vi "平均计算FRF.vi"(0 "time signal X":waveform(dbl) caption="时间信号X", 1 "restart averaging (F)":bool caption="重新开始平均(F)", 2 "window parameter":dbl=nan caption="窗参数", 5 "time signal Y":waveform(dbl) caption="时间信号Y", 7 "window":T2=1 caption="窗" items=["矩形"=0, "Hanning"=1, "Hamming"=2, "Blackman-Harris"=3, "Exact Blackman"=4, "Blackman"=5, "Flat Top"=6, "4阶Blackman-Harris "=7, "7阶Blackman-Harris"=8, "Low Sidelobe"=9, "Blackman Nuttall"=11, "三角"=30, "Bartlett-Hanning"=31, "Bohman"=32, "Parzen"=33, "Welch"=34, "Kaiser"=60, "Dolph-Chebyshev"=61, "高斯"=62], 9 "view":T1 caption="查看", 11 "error in (no error)":errorcluster caption="错误输入（无错误）", 12 "averaging parameters":T3={"averaging mode"=enum."No averaging", "weighting mode"=enum."Exponential", "number of averages"=10} caption="平均参数" {"number of averages" min=1}, 13 "FRF Mode":enum16{"H1", "H2", "H3"}(ring) caption="FRF模式", 14 "删除上一波形":bool caption="删除上一次波形") -> (3 "averaging done":bool caption="完成平均", 4 "magnitude":cluster{"f0":dbl, "df":dbl, "magnitude":dbl[]} caption="幅度" {"magnitude" format="%.2p"; "f0" format="%0.2p"; "df" format="%0.2p"}, 6 "phase":cluster{"f0":dbl, "df":dbl, "phase":dbl[]} caption="相位" {"phase" format="%.2p"; "f0" format="%0.2p"; "df" format="%0.2p"}, 8 "coherence":cluster{"f0":dbl, "df":dbl, "coherence":dbl[]} caption="相关", 10 "averages completed":dbl caption="已完成平均数" format="%.2p", 15 "error out":errorcluster caption="错误输出")   [LabVIEW 2014]
uses:
  <vilib>/Analysis/4window.llb/windowTd.ctl
  <vilib>/measure/maspectr.llb/2-chan State.ctl
  <vilib>/measure/NI_MAPro.lvlib
  <vilib>/Analysis/NI_AALPro.lvlib
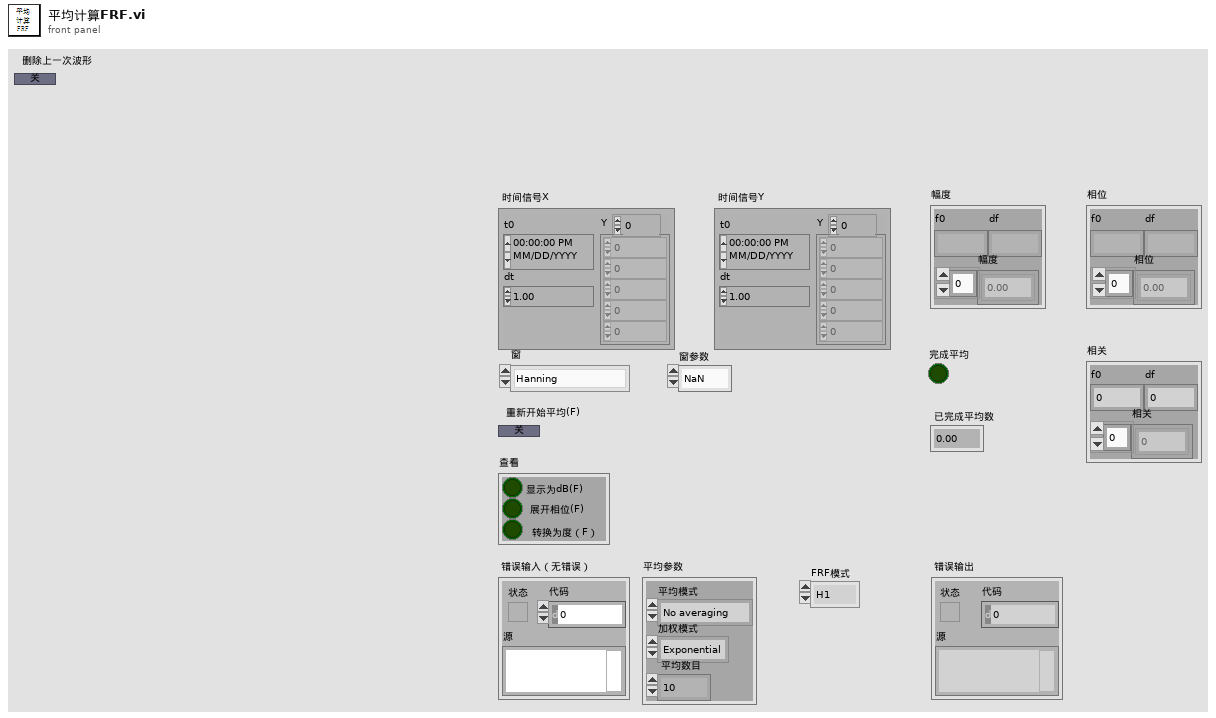
[diagram p1: front panel]
types:
  T1 = cluster{"dB On (F)":bool, "unwrap phase (F)":bool, "convert to degree (F)":bool}
  T2 = typedef "NI_AALPro.lvlib/windowTd.ctl" = u32
  T3 = cluster{"averaging mode":enum16{"No averaging", "Vector averaging", "RMS averaging", "Peak hold"}, "weighting mode":enum16{"Linear", "Exponential"}, "number of averages":u32}
  T4 = typedef "NI_MAPro.lvlib/2-chan State.ctl" = cluster{"Sx":cdb[], "Sy":cdb[], "Sxx":dbl[], "Syy":dbl[], "Sxy":cdb[], "block size":i32, "df":dbl, "dt":dbl, "avgs completed":dbl, "spectrum parameters":cluster{"averaging parameters":cluster{"averaging mode":enum16{"No averaging", "Vector averaging", "RMS averaging", "Peak hold"}, "weighting mode":enum16{"Linear", "Exponential"}, "number of averages":u32}, "window":T2}, "lin avg done":bool, "t0 history":dbl, "dt history":dbl, "timestamp":dbl}
  T5 = cluster{"f0":dbl, "df":dbl, "imag or phase":dbl[]}
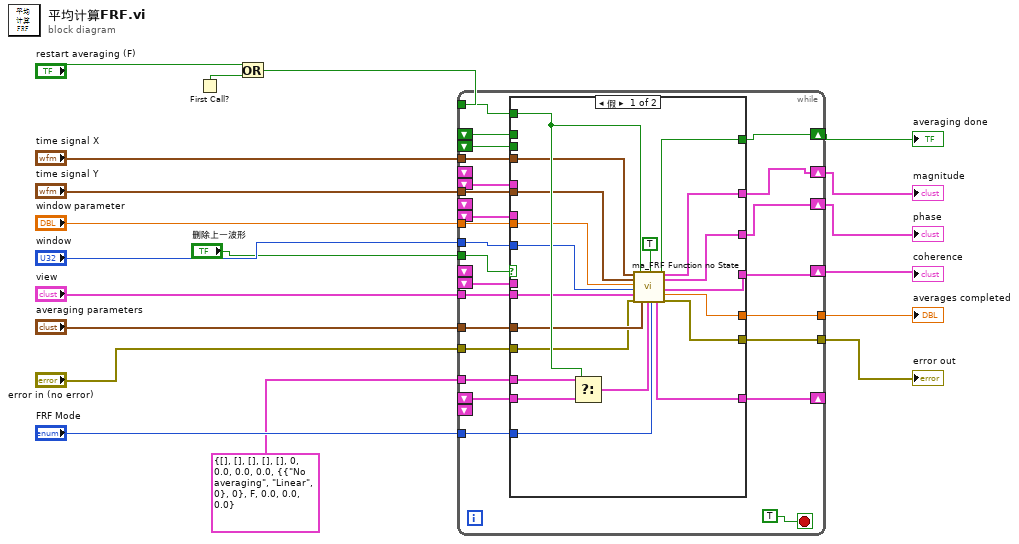
[diagram p0: block diagram]
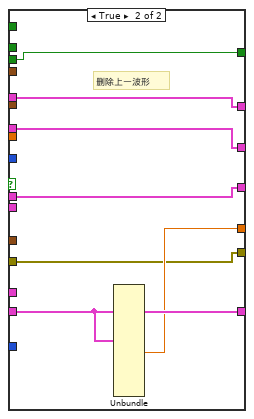
[diagram p2: hidden frame]
diagram:
  n1 = First Call?() -> (First Call?: T/F=w8:bool)
  n2 = Or(x="restart averaging (F)", y=w8) -> (x .or. y?=w6:bool)
  n3 = while {
    tunnel: w6 -> [w39]
    tunnel: [w44] -> w9
    tunnel: [w43] -> w18
    shift-right: [w42] -> _
    shift-left: _ -> [w41]
    tunnel: T4 {"Sx"=[], "Sy"=[], "Sxx"=[], "Syy"=[], "Sxy"=[], "block size"=0, "df"=0.0, "dt"=0.0, "avgs completed"=0.0, "spectrum parameters"={"averaging parameters"={"averaging mode"=enum."No averaging", "weighting mode"=enum."Linear", "number of averages"=0}, "window"=0}, "lin avg done"=FALSE, "t0 history"=0.0, "dt history"=0.0, "timestamp"=0.0} ("state info out") -> [w40]
    tunnel: "time signal X" -> [w38]
    tunnel: "time signal Y" -> [w37]
    tunnel: "window" -> [w36]
    tunnel: "view" -> [w35]
    tunnel: "averaging parameters" -> [w34]
    tunnel: "FRF Mode" -> [w33]
    tunnel: "error in (no error)" -> [w32]
    tunnel: "window parameter" -> [w31]
    shift-left: _ -> [_]
    shift-right: [w30] -> w5
    shift-left: _ -> [w29]
    shift-left: _ -> [w28]
    shift-right: [w23] -> w3
    shift-left: _ -> [_]
    shift-left: _ -> [w27]
    shift-right: [w22] -> w2
    shift-left: _ -> [_]
    shift-left: _ -> [w26]
    tunnel: "删除上一波形" -> [w25]
    shift-right: [w21] -> w1
    shift-left: _ -> [_]
    shift-left: _ -> [w24]
    stop <- TRUE stop-if-true
    n4 = case shown="假" w25 {
      tunnel: [w64 w65] -> w30
      tunnel: [w63 w70] -> w44
      tunnel: [w62 w66] -> w23
      tunnel: [w61 w69] -> w43
      tunnel: [w60 w71] -> w42
      tunnel: w41 -> [w58 w71]
      tunnel: [w56 w67] -> w22
      tunnel: w40 -> [w55 _]
      tunnel: w39 -> [w54 _]
      tunnel: w38 -> [w53 _]
      tunnel: w37 -> [w52 _]
      tunnel: w36 -> [w51 _]
      tunnel: w35 -> [w50 _]
      tunnel: w34 -> [w49 _]
      tunnel: w33 -> [w48 _]
      tunnel: [w47 w68] -> w21
      tunnel: w32 -> [w46 w69]
      tunnel: w31 -> [w45 _]
      tunnel: w29 -> [_ _]
      tunnel: w28 -> [_ w65]
      tunnel: w27 -> [_ w66]
      tunnel: w26 -> [_ w67]
      tunnel: w24 -> [_ w68]
      frame False {
        n5 = Select(t=w55, s=w54, f=w58) -> (s? t:f=w59:T4)
        n6 = call <vilib>:"ma_FRF Function no State.vi"("time signal X"=w53, "time signal Y"=w52, "window parameter"=w45, "window"=w51, "view"=w50, "error in (no error)"=w46, "restart averaging (F)"=w54, "averaging parameters"=w49, "mag-phase"=TRUE, "state info"=w59, "FRF Mode"=w48) -> ("averaging done"=w64:bool, "state info out"=w60:T4, "real or mag"=w62:cluster{"f0":dbl, "df":dbl, "real or mag":dbl[]}, "imag or phase"=w56:T5, "coherence"=w47:cluster{"f0":dbl, "df":dbl, "coherence":dbl[]}, "averages completed"=w63:dbl, "error out"=w61:errorcluster)  [unwired: 2 out]
      }
      frame True {
        # "删除上一波形"
        n7 = Unbundle ("解除捆绑")(w71) -> ("avgs completed"=w70:dbl)  [unwired: 13 out]
      }
    }
  }
  "error out" <- w18
  "averages completed" <- w9
  "averaging done" <- w5
  "coherence" <- w1
  "magnitude" <- w3
  "phase" <- w2
